vi "Sender Test.vi"() -> ()   [LabVIEW 2012]
uses:
  <vilib>/vision/NI_Vision_Development_Module.lvlib
panel:
  out "Valid Bytes Per Packet":bool
  out "Image Length":i32=8205
  in  "Image Type":T1 items=["Grayscale (U8)", "Grayscale (I16)", "Grayscale (SGL)", "Complex (CSG)", "RGB (U32)", "HSL (U32)", "RGB (U64)", "Grayscale (U16)"]
  in  "Quality (750)":i32=200
  in  "Receiver Port":u16=58432
  in  "Receiver IP Address":string="127.0.0.1"
  in  "Sender Port":u16=58432
  in  "stop":bool
  out "Image Out":T2(plugin-control)
  in  "File Path":path=path "C:/Program Files (x86)/National Instruments/Vision/Examples/Images/Blister"
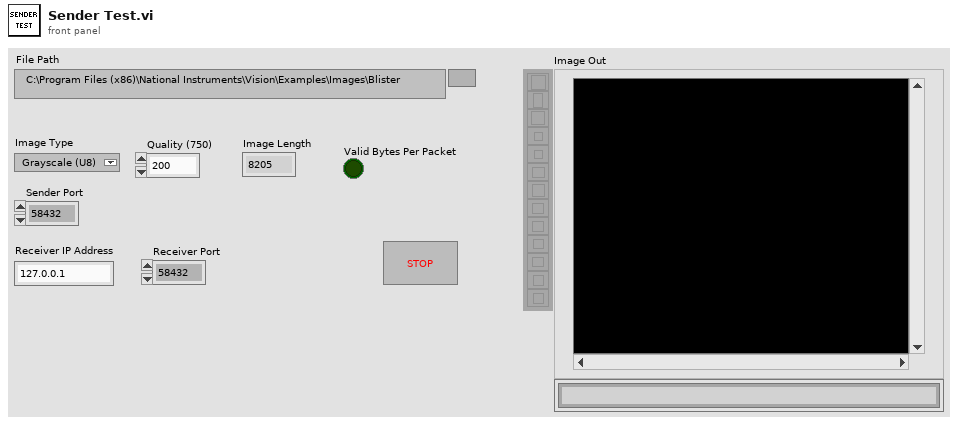
[diagram p1: front panel]
types:
  T1 = typedef "Image Type" = u32
  T2 = typedef "IMAQ Image.ctl" = refnum<image>
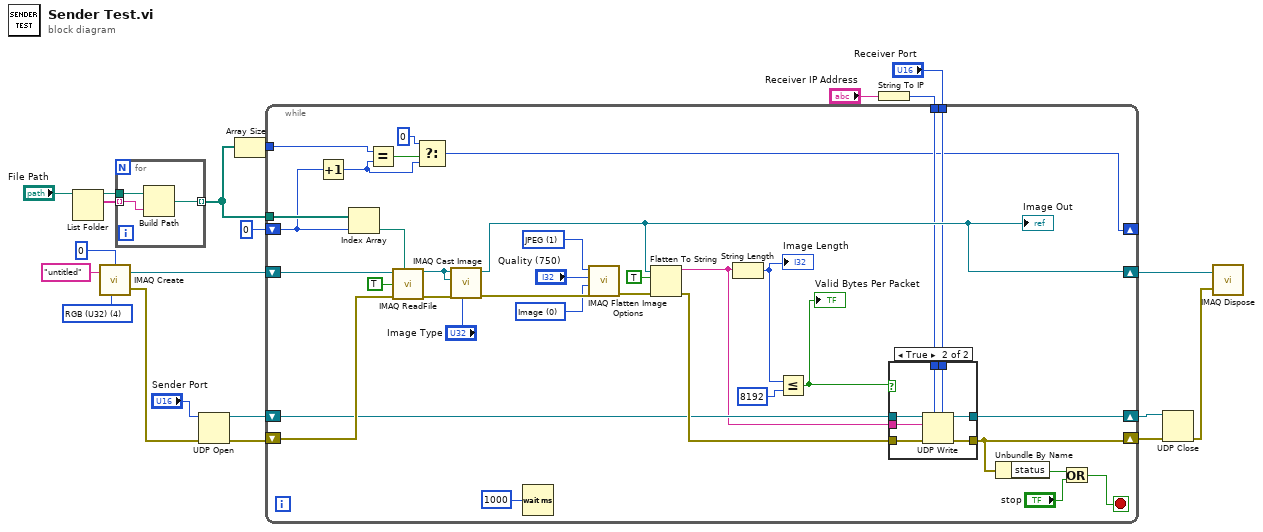
[diagram p0: block diagram]
diagram:
  w14 = T1 4 items=["Grayscale (U8)", "Grayscale (I16)", "Grayscale (SGL)", "Complex (CSG)", "RGB (U32)", "HSL (U32)", "RGB (U64)", "Grayscale (U16)"] ("Image Type 2")
  n1 = List Folder(path="File Path") -> (path out=w20:path, filenames=w19:string[])  [unwired: 3 in, 2 out]
  n2 = call "IMAQ Create"("Border Size"=0, "Image Name"="untitled", "Image Type"=w14) -> ("New Image"=w11:T2, "error out"=w10:errorcluster)  [unwired: 2 in]
  n3 = for {
    tunnel: w20 -> [w24]
    tunnel: w19 -> [w23] mode=indexing
    tunnel: [w22] -> w8 mode=indexing
    n4 = Build Path(base path=w24, name or relative path=w23) -> (appended path=w22:path)
  }
  n5 = UDP Open(8:w10, 11:"Sender Port") -> (port=w16:refnum<k16>, 0:w17:errorcluster)  [unwired: 3 in, 1 out]
  n6 = Array Size(array=w8) -> (size(s)=w15:i32)
  n7 = String To IP(1:"Receiver IP Address") -> (0:w1:u32)
  n8 = while {
    tunnel: w15 -> [w35]
    tunnel: w8 -> [w56]
    shift-right: [w31] -> _
    shift-left: 0 ("index") -> [w36]
    shift-right: [w47] -> w7
    shift-left: w11 -> [w57]
    shift-right: [w28] -> w6
    shift-left: w17 -> [w58]
    shift-right: [w41] -> w5
    shift-left: w16 -> [w44]
    tunnel: "Receiver Port" -> [w38]
    tunnel: w1 -> [w37]
    stop <- w27 stop-if-true
    w49 = 0 items=["Image", "Image and Vision Info", "Reference to Image"] ("Type of Flatten (Image and Vision Info)")
    w51 = 1 items=["None", "JPEG", "PACKED BINARY"] ("Compression (None)")
    n9 = Increment(x=w36) -> (x+1=w32:i32)
    n10 = Index Array(array=w56, index=w36) -> (element=w55:path)
    n11 = Equal?(x=w35, y=w32) -> (x = y?=w34:bool)
    n12 = call "IMAQ ReadFile"("File Path"=w55, "error in (no error)"=w58, "Load Color Palette? (No)"=TRUE, "Image"=w57) -> ("error out"=w54:errorcluster, "Image Out"=w53:T2)  [unwired: 3 in, 3 out]
    n13 = Select(t=0 ("index"), s=w34, f=w32) -> (s? t:f=w31:i32)
    n14 = call "IMAQ Cast Image"("Image Type"="Image Type", "error in (no error)"=w54, "Image Dst"=w53, "Image Src"=w53) -> ("error out"=w52:errorcluster, "Image Dst Out"=w47:T2)  [unwired: 6 in]
    "Image Out" <- w47
    n15 = Wait (ms)(milliseconds to wait=u32 1000) -> ()  [unwired: 1 out]
    n16 = call "IMAQ Flatten Image Options"("error in (no error)"=w52, "Type of Flatten (Image and Vision Info)"=w49, "Quality (750)"="Quality (750)", "Compression (None)"=w51) -> ("error out"=w48:errorcluster)  [unwired: 4 in, 3 out]
    n17 = Flatten To String(anything=w47, prepend array or string size? (T)=TRUE, error in (no error)=w48) -> (data string=w40:string, error out=w45:errorcluster)  [unwired: 1 in, 1 out]
    n18 = String Length(string=w40) -> (length=w39:i32)
    "Image Length" <- w39
    n19 = Less Or Equal?(x=w39, y=8192) -> (x <= y?=w26:bool)
    "Valid Bytes Per Packet" <- w26
    n20 = case shown="True" w26 {
      tunnel: w45 -> [w61 w68]
      tunnel: w44 -> [w60 w67]
      tunnel: [w61 w66] -> w28
      tunnel: [w60 w65] -> w41
      tunnel: w40 -> [_ w64]
      tunnel: w38 -> [_ w63]
      tunnel: w37 -> [_ w62]
      frame False {
      }
      frame True {
        n21 = UDP Write(address=w62, port or service name=w63, connection ID=w67, data in=w64, 8:w68) -> (error out=w66:errorcluster, 3:w65:refnum<k16>)  [unwired: 1 in]
      }
    }
    n22 = Unbundle By Name(w28) -> ("status"=w29:bool)
    n23 = Or(x=w29, y="stop") -> (x .or. y?=w27:bool)
  }
  n24 = UDP Close(connection ID=w5, 8:w6) -> (error out=w4:errorcluster)  [unwired: 1 out]
  n25 = call "IMAQ Dispose"("Image"=w7, "error in (no error)"=w4) -> ()  [unwired: 4 in, 1 out]
